vi "emi_Get VI ref if missing.vi"(5 "VI Refnum(This VI)":refnum<vi>, 9 "error in (no error)":errorcluster) -> (2 "Ref Generated":bool=TRUE, 6 "VI Refnum Out":refnum<vi>, 10 "error out":errorcluster)   [LabVIEW 2010]
doc: "If VI Refnumis connected to a valid ref number, nothing is done. If it is not, the refnumber of the Current VI is returned. \n\nThe Idee: help making VIs that default to working with the VI they are placed on. \n\nNo ref number is created if error in."
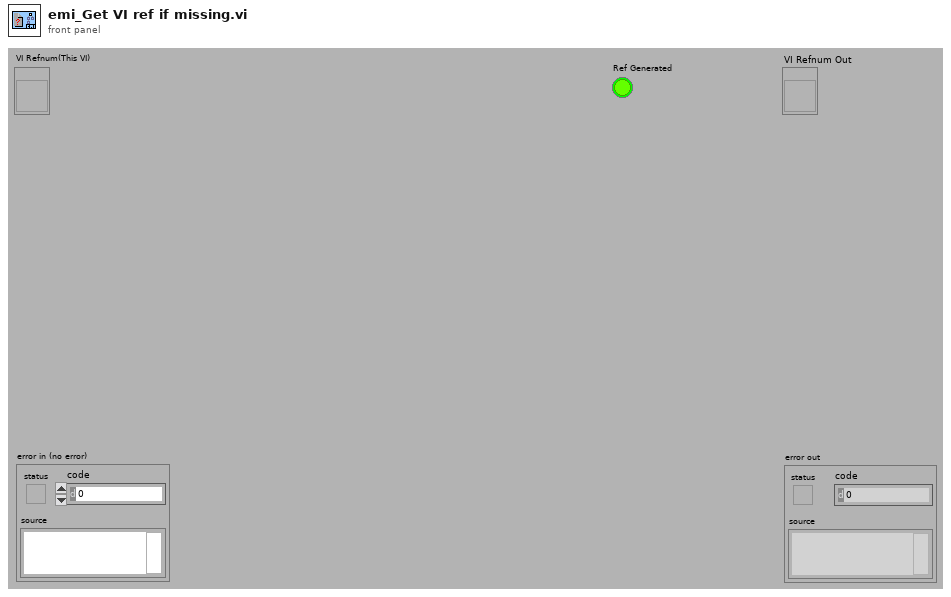
[diagram p1: front panel]
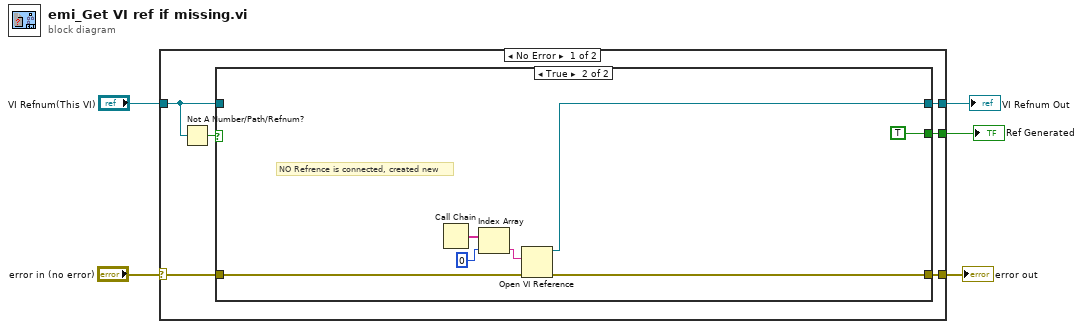
[diagram p0: block diagram]
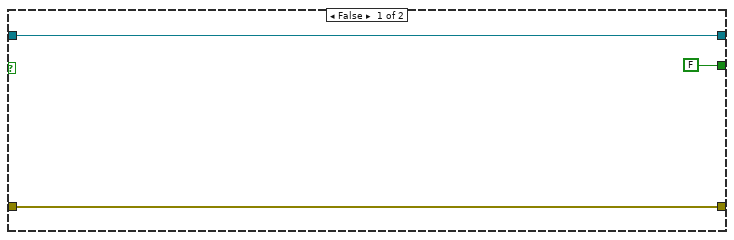
[diagram p2: hidden frame]
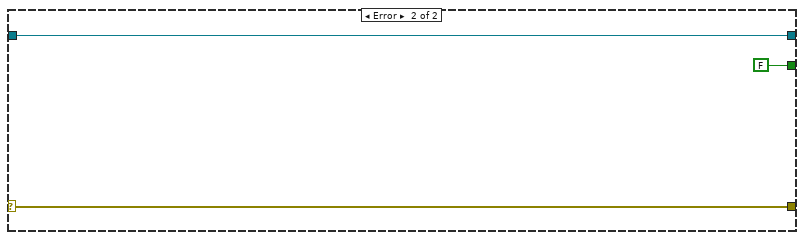
[diagram p3: hidden frame]
diagram:
  n1 = case shown="No Error" "error in (no error)" {
    selector: "error in (no error)" -> [w7 w24]
    tunnel: [w11 w24] -> w5
    tunnel: [w10 w23] -> w4
    tunnel: "VI Refnum(This VI)" -> [w8 w23]
    tunnel: [w6 FALSE ("Ref Generated")] -> w1
    frame No Error {
      n2 = Not A Number/Path/Refnum?(number/path/refnum=w8) -> (NaN/Path/Refnum?=w9:bool)
      n3 = case shown="True" w9 {
        tunnel: [w13 w15] -> w11
        tunnel: [w14 w18] -> w10
        tunnel: w8 -> [w14 _]
        tunnel: w7 -> [w13 w16]
        tunnel: [FALSE ("Ref Generated") TRUE ("Ref Generated")] -> w6
        frame False {
        }
        frame True {
          # "NO Refrence is connected, created new"
          n4 = Call Chain() -> (call chain=w21:string[])
          n5 = Index Array(array=w21, index=0) -> (element=w19:string)
          n6 = Open VI Reference(vi path=w19, error in (no error)=w16) -> (vi reference=w18:refnum<vi>, error out=w15:errorcluster)  [unwired: 4 in]
        }
      }
    }
    frame Error {
    }
  }
  "error out" <- w5
  "Ref Generated" <- w1
  "VI Refnum Out" <- w4
